vi "SQL查询.vi"(7 "condition":string, 8 "error in (no error)":errorcluster, 9 "columns":string[](array[string]), 10 "table输入":string(combo), 11 "database":string(combo)) -> (0 "error out":errorcluster, 1 "拆分数据":bool, 2 "columns输出":string[](array[string]), 3 "data":string[][](table))   [LabVIEW 2016, in "数据传输系统.lvlib"]
uses:
  <vilib>/Utility/sysdir.llb/System Directory Type.ctl
  <vilib>/addons/database/Connection.llb/DB Tools Open Connec (String).vi
  <vilib>/addons/database/_DB Variant To Data/Database Variant To Data.xnode
  <vilib>/addons/database/NI_Database_API.lvlib
panel:
  out "元素":string
  out "子数组":string[](array[string])
  # "时间 > #2021/01/15 08:00:00#and 时间 < #2021/04/15 08:00:00# order by 时间 asc"
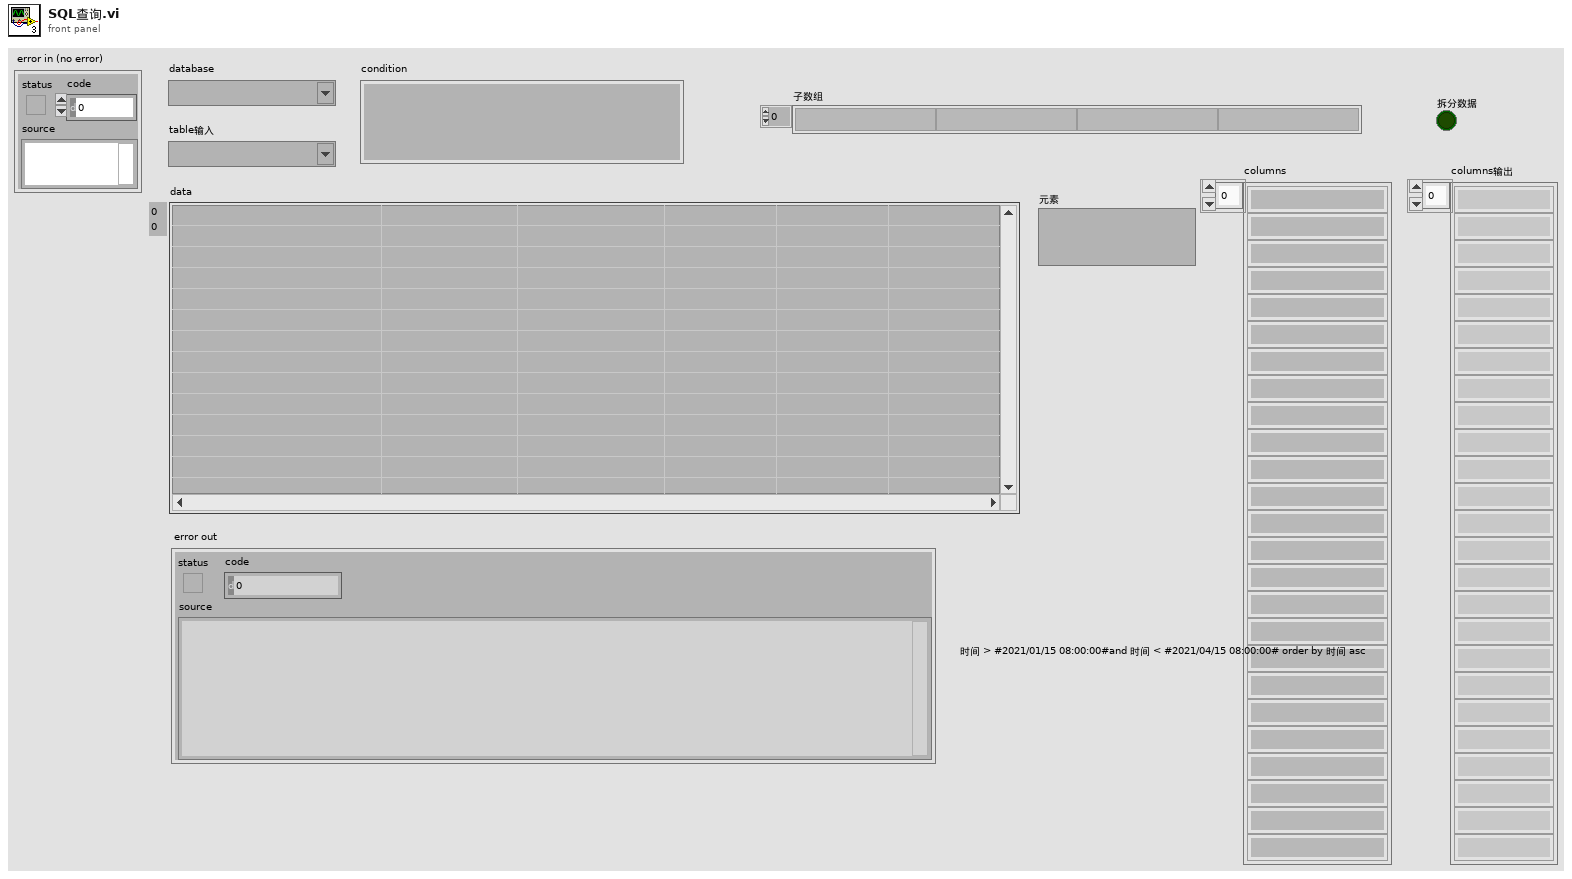
[diagram p1: front panel]
types:
  T1 = typedef "System Directory Type.ctl" = i32
  T2 = typedef "NI_Database_API.lvlib/Conn ObjectReference.ctl" = refnum<k1>
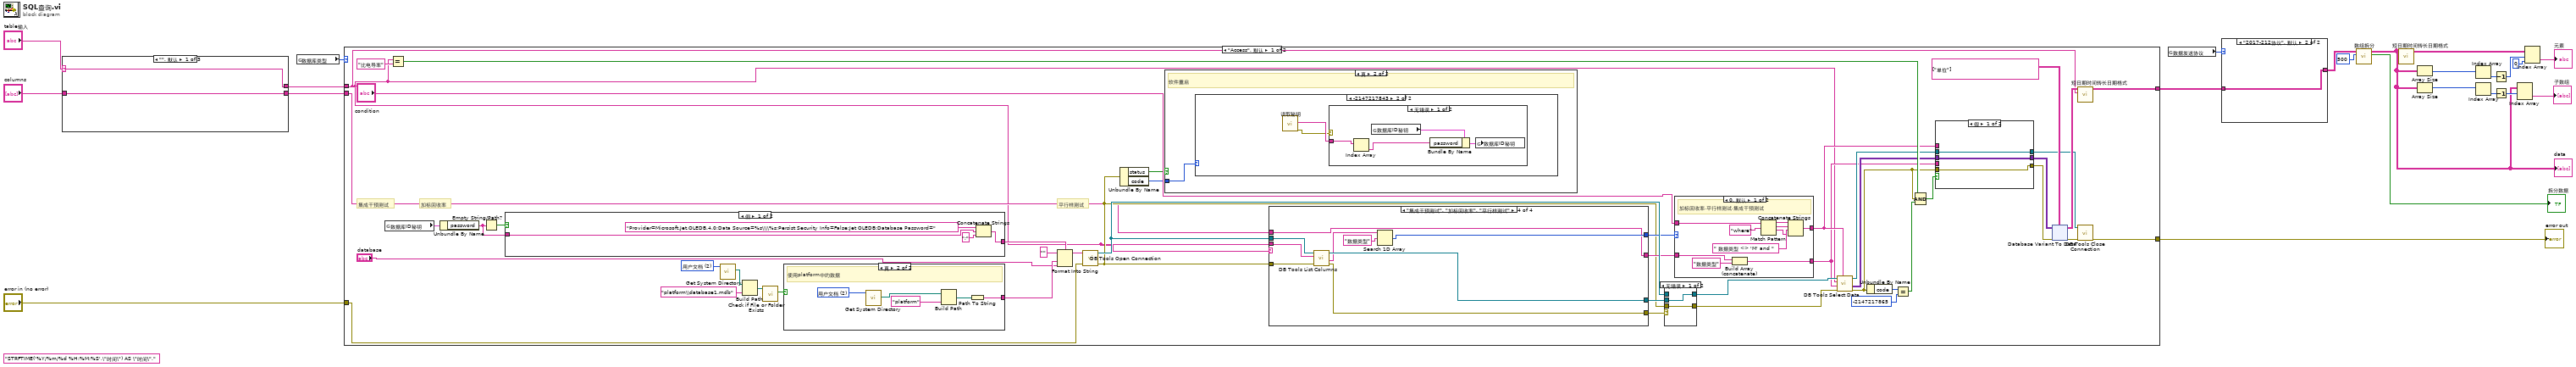
[diagram p0: block diagram]
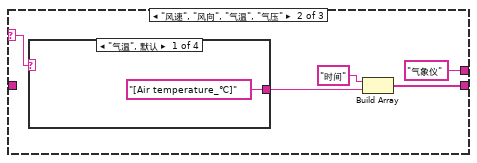
[diagram p2: hidden frame]
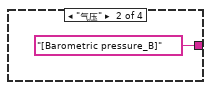
[diagram p3: hidden frame]
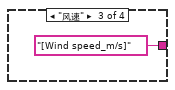
[diagram p4: hidden frame]
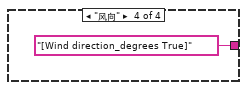
[diagram p5: hidden frame]
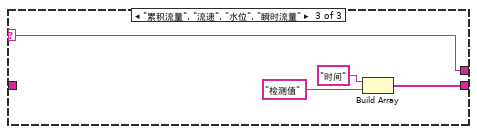
[diagram p6: hidden frame]
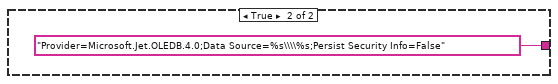
[diagram p7: hidden frame]
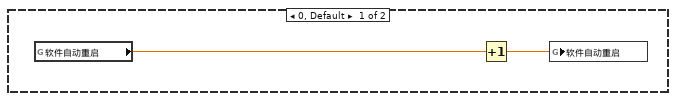
[diagram p9: hidden frame]
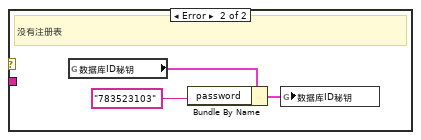
[diagram p10: hidden frame]
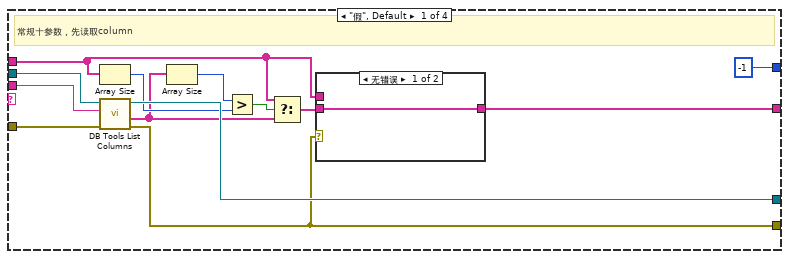
[diagram p13: hidden frame]
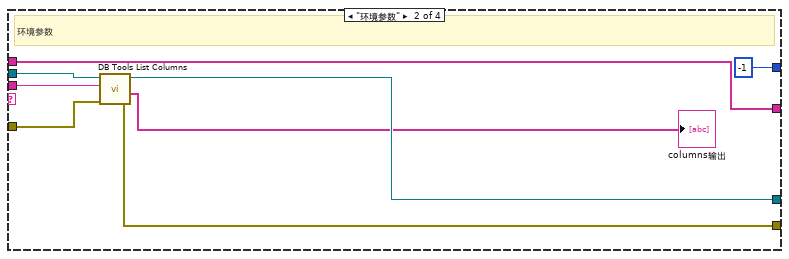
[diagram p15: hidden frame]
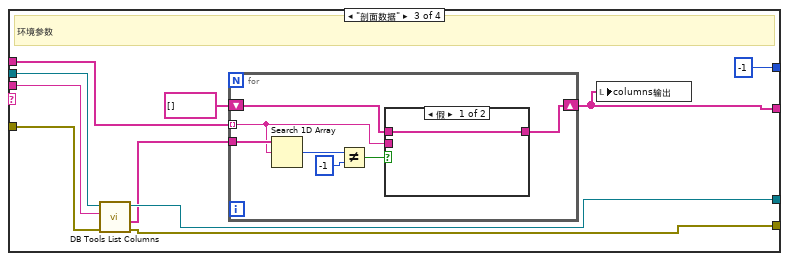
[diagram p16: hidden frame]
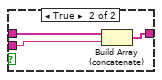
[diagram p17: hidden frame]
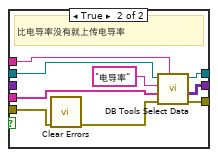
[diagram p18: hidden frame]
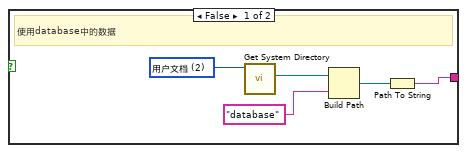
[diagram p19: hidden frame]
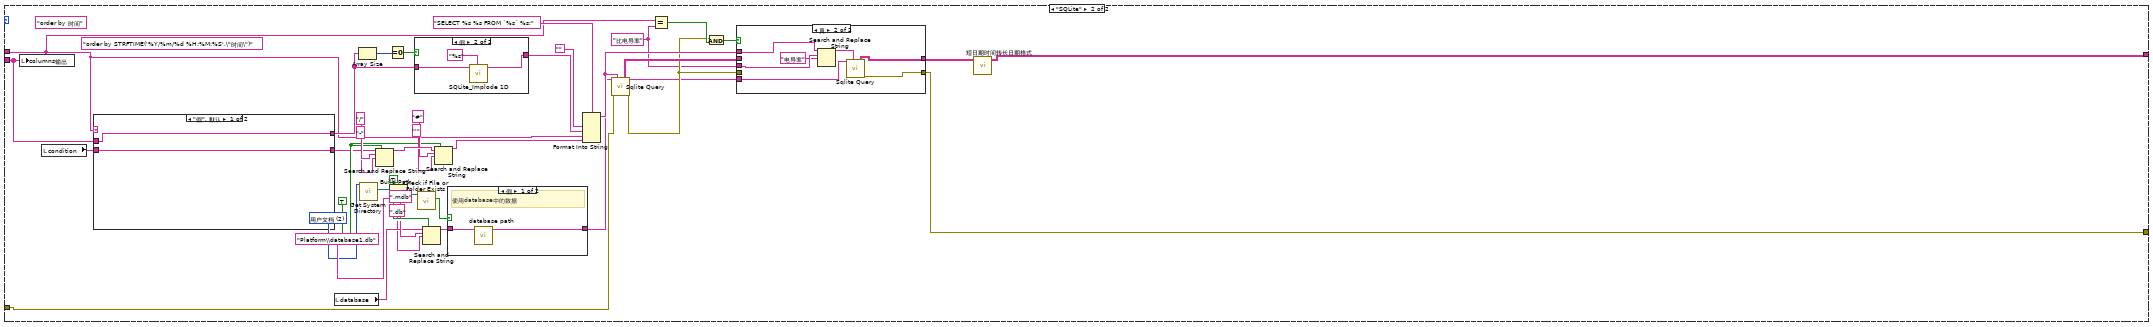
[diagram p20: hidden frame]
diagram:
  (unwired) "STRFTIME('%Y/%m/%d %H:%M:%S',\"时间\") AS \"时间\"," ("输入 1")
  n1 = case shown="\"\", 默认" "table输入" {
    selector: "table输入" -> [w25 w29 w35]
    tunnel: [w25 "气象仪" w35] -> w4
    tunnel: "columns" -> [w24 _ _]
    tunnel: [w24 w26 w37] -> w5
    frame "", Default {
    }
    frame "风速", "风向", "气温", "气压" {
      n2 = case shown="\"气温\", 默认" w29 {
        tunnel: ["[Air temperature_℃]" "[Barometric pressure_B]" "[Wind speed_m/s]" "[Wind direction_degrees True]"] -> w27
        frame "气温", Default {
        }
        frame "气压" {
        }
        frame "风速" {
        }
        frame "风向" {
        }
      }
      n3 = Build Array("时间", w27) -> (w26:string[])
    }
    frame "累积流量", "流速", "水位", "瞬时流量" {
      n4 = Build Array("时间", "检测值") -> (w37:string[])
    }
  }
  n5 = global read "断电保存全局.vi" "数据库类型"() -> (w8:enum16{"Access", "SQLite"})
  n6 = case shown="\"Access\", 默认" w8 {
    tunnel: [w79 w270] -> w23
    tunnel: [w51 w246] -> w11
    tunnel: "error in (no error)" -> [w43 w239]
    tunnel: w5 -> [w41 w242]
    tunnel: w4 -> [w40 w241]
    frame "Access", Default {
      w77 = T1 2 items=["用户目录"=0, "用户桌面"=1, "用户文档"=2, "用户应用程序数据"=3, "用户设置"=4, "用户临时目录"=5, "公共文档"=6, "公共应用程序数据"=7, "公共设置"=8, "公共缓存"=13, "系统核心库"=9, "系统安装库"=10, "应用程序文件"=11, "启动盘根目录"=12] ("system directory type")
      # "集成干预测试"
      # "平行样测试"
      # "加标回收率"
      n7 = global read "外部交互全局.vi" "数据库ID秘钥"() -> (w44:cluster{"userID":string, "password":string})
      n8 = Equal?(x=w40, y="比电导率") -> (x = y?=w71:bool)
      n9 = Unbundle By Name(w44) -> ("password"=w45:string)
      n10 = Empty String/Path?(string/path=w45) -> (empty?=w47:bool)
      n11 = case shown="假" w47 {
        tunnel: [w85 "Provider=Microsoft.Jet.OLEDB.4.0;Data Source=%s\\\\%s;Persist Security Info=False" ("格式字符串")] -> w46
        tunnel: w45 -> [w88 _]
        frame False {
          n12 = Concatenate Strings("Provider=Microsoft.Jet.OLEDB.4.0;Data Source=%s\\\\%s;Persist Security Info=False;Jet OLEDB:Database Password=" ("格式字符串"), w88, ";" ("字符串")) -> (w85:string)
        }
        frame True {
        }
      }
      n13 = call <vilib>:"Get System Directory.vi"("system directory type"=w77) -> ("system directory"=w78:path)  [unwired: 10 in]
      n14 = Build Path(base path=w78, name or relative path="platform\\database1.mdb" ("condition")) -> (appended path=w76:path)
      n15 = call <vilib>:"Check if File or Folder Exists.vi"("path"=w76) -> ("file or folder exists?"=w74:bool)  [unwired: 8 in, 2 out]
      n16 = case shown="真" w74 {
        tunnel: [w183 w188] -> w73
        frame False {
          w186 = T1 2 items=["用户目录"=0, "用户桌面"=1, "用户文档"=2, "用户应用程序数据"=3, "用户设置"=4, "用户临时目录"=5, "公共文档"=6, "公共应用程序数据"=7, "公共设置"=8, "公共缓存"=13, "系统核心库"=9, "系统安装库"=10, "应用程序文件"=11, "启动盘根目录"=12] ("system directory type")
          # "使用database中的数据"
          n17 = call <vilib>:"Get System Directory.vi"("system directory type"=w186) -> ("system directory"=w185:path)  [unwired: 10 in]
          n18 = Build Path(base path=w185, name or relative path="database" ("condition")) -> (appended path=w187:path)
          n19 = Path To String(path=w187) -> (string=w183:string)
        }
        frame True {
          w192 = T1 2 items=["用户目录"=0, "用户桌面"=1, "用户文档"=2, "用户应用程序数据"=3, "用户设置"=4, "用户临时目录"=5, "公共文档"=6, "公共应用程序数据"=7, "公共设置"=8, "公共缓存"=13, "系统核心库"=9, "系统安装库"=10, "应用程序文件"=11, "启动盘根目录"=12] ("system directory type")
          # "使用platform中的数据"
          n20 = call <vilib>:"Get System Directory.vi"("system directory type"=w192) -> ("system directory"=w191:path)  [unwired: 10 in]
          n21 = Build Path(base path=w191, name or relative path="platform" ("condition")) -> (appended path=w189:path)
          n22 = Path To String(path=w189) -> (string=w188:string)
        }
      }
      n23 = Format Into String(format string=w46, initial string="" ("初始字符串"), w73, "database") -> (resulting string=w81:string)  [unwired: 1 in, 1 out]
      n24 = call-poly <vilib>:"DB Tools Open Connection.vi"("error in (no error)"=w43, "connection information"=w81) -> ("error out"=w52:errorcluster, "connection reference"=w57:T2)  [unwired: 6 in]
      n25 = Unbundle By Name(w52) -> ("status"=w50:bool, "code"=w39:i32)
      n26 = case shown="真" w50 {
        tunnel: w39 -> [_ w90]
        frame False {
        }
        frame True {
          # "软件重启"
          n27 = case shown="-2147217843" w90 {
            frame 0, Default {
              n28 = global read "全局1.vi" "软件自动重启"() -> (w92:dbl)
              n29 = Increment(x=w92) -> (x+1=w91:dbl)
              n30 = global write "全局1.vi" "软件自动重启"(w91) -> ()
            }
            frame -2147217843 {
              n31 = call "读取秘钥.vi"() -> ("error out"=w93:errorcluster, "值"=w94:string[])  [unwired: 9 in, 1 out]
              n32 = case shown="无错误" w93 {
                tunnel: w94 -> [w98 _]
                frame No Error {
                  n33 = Index Array(array=w98) -> (element=w95:string)  [unwired: 1 in]
                  n34 = global read "外部交互全局.vi" "数据库ID秘钥"() -> (w96:cluster{"userID":string, "password":string})
                  n35 = Bundle By Name(cluster=w96, "password"=w95) -> (w97:cluster{"userID":string, "password":string})
                  n36 = global write "外部交互全局.vi" "数据库ID秘钥"(w97) -> ()
                }
                frame Error {
                  # "没有注册表"
                  n37 = global read "外部交互全局.vi" "数据库ID秘钥"() -> (w100:cluster{"userID":string, "password":string})
                  n38 = Bundle By Name(cluster=w100, "password"="783523103") -> (w101:cluster{"userID":string, "password":string})
                  n39 = global write "外部交互全局.vi" "数据库ID秘钥"(w101) -> ()
                }
              }
            }
          }
        }
      }
      n40 = case shown="\"集成干预测试\", \"加标回收率\", \"平行样测试\"" w40 {
        tunnel: w57 -> [w129 w140 w148 w170]
        tunnel: w52 -> [w126 w139 w147 w168]
        tunnel: [w127 w138 w145 w167] -> w59
        tunnel: [w121 w137 w146 w166] -> w60
        tunnel: w40 -> [w128 w136 w149 w169]
        tunnel: [-1 ("index of element") -1 ("index of element") -1 ("index of element") w163] -> w55
        tunnel: w41 -> [w118 w133 w144 w162]
        tunnel: [w119 w133 w141 w162] -> w53
        frame "假", Default {
          # "常规十参数，先读取column"
          n41 = Array Size(array=w118) -> (size(s)=w123:i32)
          n42 = call <vilib>:"DB Tools List Columns.vi"("error in (no error)"=w126, "table"=w128, "connection reference"=w129) -> ("error out"=w121:errorcluster, "columns"=w122:string[], "connection reference out"=w127:T2)  [unwired: 1 in, 1 out]
          n43 = Array Size(array=w122) -> (size(s)=w124:i32)
          n44 = Greater?(x=w124, y=w123) -> (0:w125:bool)
          n45 = Select(t=w118, s=w125, f=w122) -> (s? t:f=w120:string[])
          n46 = case shown="无错误" w121 {
            tunnel: w120 -> [w131 _]
            tunnel: [w131 w132] -> w119
            tunnel: w118 -> [_ w132]
            frame No Error {
            }
            frame Error {
            }
          }
        }
        frame "环境参数" {
          # "环境参数"
          n47 = call <vilib>:"DB Tools List Columns.vi"("error in (no error)"=w139, "table"=w136, "connection reference"=w140) -> ("error out"=w137:errorcluster, "columns"=→"columns输出":string[], "connection reference out"=w138:T2)  [unwired: 1 in, 1 out]
        }
        frame "剖面数据" {
          # "环境参数"
          n48 = call <vilib>:"DB Tools List Columns.vi"("error in (no error)"=w147, "table"=w149, "connection reference"=w148) -> ("error out"=w146:errorcluster, "columns"=w143:string[], "connection reference out"=w145:T2)  [unwired: 1 in, 1 out]
          n49 = for {
            tunnel: w144 -> [w153] mode=indexing
            tunnel: w143 -> [w157]
            shift-right: [w151] -> w141
            shift-left: string[] [] -> [w154]
            n50 = Search 1D Array(1D array=w157, element=w153) -> (index of element=w156:i32)  [unwired: 1 in]
            n51 = Not Equal?(x=w156, y=-1) -> (x != y?=w152:bool)
            n52 = case shown="假" w152 {
              tunnel: w154 -> [w158 w161]
              tunnel: w153 -> [_ w160]
              tunnel: [w158 w159] -> w151
              frame False {
              }
              frame True {
                n53 = Build Array (concatenate)(w161, w160) -> (w159:string[])
              }
            }
          }
          n54 = local write "columns输出"(w141) -> ()
        }
        frame "集成干预测试", "加标回收率", "平行样测试" {
          n55 = call <vilib>:"DB Tools List Columns.vi"("error in (no error)"=w168, "table"=w169, "connection reference"=w170) -> ("error out"=w166:errorcluster, "columns"=w165:string[], "connection reference out"=w167:T2)  [unwired: 1 in, 1 out]
          n56 = Search 1D Array(1D array=w165, element="数据类型" ("元素")) -> (index of element=w163:i32)  [unwired: 1 in]
        }
      }
      n57 = case shown="无错误" w60 {
        selector: w60 -> [_ w117]
        tunnel: w59 -> [w115 _]
        tunnel: [w115 w116] -> w58
        tunnel: w57 -> [_ w116]
        tunnel: [w114 w117] -> w56
        tunnel: w52 -> [w114 _]
        frame No Error {
        }
        frame Error {
        }
      }
      n58 = case "条件结构" shown="0, 默认" w55 {
        tunnel: "condition" -> [w109 w112]
        tunnel: w53 -> [w111 w113]
        tunnel: [w103 w113] -> w48
        tunnel: [w102 w112] -> w49
        frame 0, Default {
          # "加标回收率,平行样测试,集成干预测试"
          n59 = Build Array (concatenate)(w111, "数据类型" ("元素")) -> (w103:string[])
          n60 = Match Pattern(string=w109, regular expression="where" ("正则表达式")) -> (before substring=w107:string, match substring=w106:string, after substring=w104:string)  [unwired: 1 in, 1 out]
          n61 = Concatenate Strings(w107, w106, " 数据类型 <> 'M' and " ("字符串"), w104) -> (w102:string)
        }
        frame -1 {
        }
      }
      n62 = call <vilib>:"DB Tools Select Data.vi"("condition"=w49, "error in (no error)"=w56, "columns"=w48, "table"=w40, "connection reference"=w58) -> ("error out"=w64:errorcluster, "data"=w66:variant[][], "connection reference out"=w69:T2)  [unwired: 1 in]
      n63 = Unbundle By Name(w64) -> ("code"=w63:i32)
      n64 = Equal?(x=w63, y=-2147217865 ("code")) -> (x = y?=w61:bool)
      n65 = Compound Arithmetic op=AND ("复合运算")(w71, w64, w61) -> (w70:bool)
      n66 = case shown="假" w70 {
        tunnel: w49 -> [_ w182]
        tunnel: w69 -> [w173 w181]
        tunnel: [w173 w176] -> w68
        tunnel: [w172 w177] -> w67
        tunnel: w66 -> [w172 _]
        tunnel: w64 -> [w171 w179]
        tunnel: [w171 w175] -> w65
        tunnel: w48 -> [_ w174]
        frame False {
        }
        frame True {
          # "比电导率没有就上传电导率"
          n67 = call <vilib>:"Clear Errors.vi"("error in (no error)"=w179) -> ("error out"=w178:errorcluster)  [unwired: 5 in, 1 out]
          n68 = call <vilib>:"DB Tools Select Data.vi"("condition"=w182, "error in (no error)"=w178, "columns"=w174, "table"="电导率", "connection reference"=w181) -> ("error out"=w175:errorcluster, "data"=w177:variant[][], "connection reference out"=w176:T2)  [unwired: 1 in]
        }
      }
      n69 = xnode "Database Variant To Data"("database variant"=w67, "error in (no error)"=w65, "type"=string[][] [["单位"]]) -> ("data"=w80:string[][], "error out"=w82:errorcluster)
      n70 = call "短日期时间转长日期格式.vi"("table输入"=w40, "data"=w80) -> ("输出数组"=w79:string[][])  [unwired: 9 in]
      n71 = call <vilib>:"DB Tools Close Connection.vi"("error in (no error)"=w82, "connection reference"=w68) -> ("error out"=w51:errorcluster)  [unwired: 5 in]
    }
    frame "SQLite" {
      w244 = "比电导率" ("y")
      (unwired) "order by STRFTIME('%Y/%m/%d %H:%M:%S',\"时间\")" ("替换字符串(\"\")")
      (unwired) "order by 时间" ("搜索字符串")
      w255 = TRUE ("替换全部？(F)")
      w272 = T1 2 items=["用户目录"=0, "用户桌面"=1, "用户文档"=2, "用户应用程序数据"=3, "用户设置"=4, "用户临时目录"=5, "公共文档"=6, "公共应用程序数据"=7, "公共设置"=8, "公共缓存"=13, "系统核心库"=9, "系统安装库"=10, "应用程序文件"=11, "启动盘根目录"=12] ("system directory type")
      n72 = local write "columns输出"(w242) -> ()
      n73 = local read "condition"() -> (w254:string)
      n74 = case shown="\"假\", 默认" w241 {
        tunnel: w254 -> [w286 w292]
        tunnel: w242 -> [w285 w294]
        tunnel: [w285 w293] -> w265
        tunnel: [w286 w291] -> w253
        frame "假", Default {
        }
        frame "集成干预测试", "加标回收率", "平行样测试" {
          n75 = Build Array (concatenate)(w294, "数据类型" ("元素")) -> (w293:string[])
          n76 = call "数据库加密匹配 (子VI).vi"("输入参数"="N") -> ("Encoded String"=w289:string)  [unwired: 10 in]
          n77 = Match Pattern(string=w292, regular expression="where" ("正则表达式")) -> (before substring=w297:string, match substring=w296:string, after substring=w295:string)  [unwired: 1 in, 1 out]
          n78 = Format Into String(format string=" 数据类型 = '%s' and " ("字符串"), w289) -> (resulting string=w287:string)  [unwired: 2 in, 1 out]
          n79 = Concatenate Strings(w297, w296, w287, w295) -> (w291:string)
        }
      }
      n80 = local read "database"() -> (w257:string)
      n81 = Array Size(array=w265) -> (size(s)=w269:i32)
      n82 = call <vilib>:"Get System Directory.vi"("system directory type"=w272) -> ("system directory"=w271:path)  [unwired: 10 in]
      n83 = Search and Replace String(replace all?=w255, input string=w253, search string="/" ("搜索字符串"), replace string="-" ("替换字符串(\"\")")) -> (result string=w262:string)  [unwired: 4 in, 3 out]
      n84 = Equal To 0?(x=w269) -> (x = 0?=w268:bool)
      n85 = Build Path(base path=w271, name or relative path="Platform\\database1.db" ("condition")) -> (appended path=w273:path)
      n86 = case shown="假" w268 {
        tunnel: w265 -> [_ w302]
        tunnel: ["*" ("t") w301] -> w266
        frame True {
        }
        frame False {
          n87 = call <userlib>:"SQLite_Implode 1D.vi"("Values"=w302, "format string"="%s") -> ("imploded string"=w301:string)  [unwired: 7 in, 1 out]
        }
      }
      n88 = call <vilib>:"Check if File or Folder Exists.vi"("path"=w273) -> ("file or folder exists?"=w275:bool)  [unwired: 8 in, 2 out]
      n89 = Search and Replace String(replace all?=TRUE ("替换全部？(F)"), input string=w257, search string=".mdb" ("搜索字符串"), replace string=".db" ("替换字符串(\"\")")) -> (result string=w252:string)  [unwired: 4 in, 3 out]
      n90 = Search and Replace String(replace all?=w255, input string=w262, search string="#" ("搜索字符串"), replace string="'" ("替换字符串(\"\")")) -> (result string=w237:string)  [unwired: 4 in, 3 out]
      n91 = case shown="假" w275 {
        tunnel: [w305 w306] -> w240
        tunnel: w252 -> [w304 w307]
        frame False {
          # "使用database中的数据"
          n92 = call "database path.vi"("database"=w304) -> ("Path out"=w305:string)  [unwired: 9 in, 1 out]
        }
        frame True {
          # "使用platform中的数据"
          n93 = call "database platform path.vi"("database"=w307) -> ("Path out"=w306:string)  [unwired: 10 in]
        }
      }
      n94 = Format Into String(format string="SELECT %s %s FROM `%s` %s;" ("SQL Query"), "", w266, w241, w237) -> (resulting string=w247:string)  [unwired: 2 in, 1 out]
      n95 = call "Sqlite Query.vi"("DB Path"=w240, "SQL Query"=w247, "error in (no error)"=w239) -> ("Results"=w249:string[][], "DB Path Out"=w243:string, "error out"=w245:errorcluster)  [unwired: 10 in]
      n96 = Equal?(x=w241, y=w244) -> (x = y?=w251:bool)
      n97 = And(x=w245, y=w251) -> (x .and. y?=w250:bool)
      n98 = case shown="真" w250 {
        tunnel: w249 -> [w277 _]
        tunnel: [w277 w284] -> w248
        tunnel: w247 -> [_ w281]
        tunnel: w243 -> [_ w283]
        tunnel: [w276 w282] -> w246
        tunnel: w245 -> [w276 _]
        tunnel: w244 -> [_ w280]
        frame False {
        }
        frame True {
          n99 = Search and Replace String(input string=w281, search string=w280, replace string="电导率" ("Tables Name")) -> (result string=w278:string)  [unwired: 5 in, 3 out]
          n100 = call "Sqlite Query.vi"("DB Path"=w283, "SQL Query"=w278) -> ("Results"=w284:string[][], "error out"=w282:errorcluster)  [unwired: 11 in, 1 out]
        }
      }
      n101 = call "短日期时间转长日期格式.vi"("data"=w248) -> ("输出数组"=w270:string[][])  [unwired: 10 in]
    }
  }
  "error out" <- w11
  n102 = global read "断电保存全局.vi" "数据发送协议"() -> (w22:enum16{"2005-212协议", "2017-212协议"})
  n103 = case shown="\"2017-212协议\", 默认" w22 {
    tunnel: w23 -> [w309 w316]
    tunnel: [w308 w316] -> w9
    frame "2005-212协议" {
      n104 = for {
        N: 1 -> [_]
        tunnel: string[][] [] ("data") -> [w315]
        tunnel: w309 -> [w314] mode=indexing
        tunnel: [w312] -> w308
        n105 = Insert Into Array(array=w315, index (row)=0 ("索引 (行)"), new element=w314) -> (w312:string[][])  [unwired: 1 in]
      }
    }
    frame "2017-212协议", Default {
    }
  }
  n106 = call "数组拆分.vi"("拆分大小"=500, "输入数据"=w9) -> ("拆分数据"=→"拆分数据":bool, "输出数组"=w1:string[][])  [unwired: 8 in]
  "data" <- w1
  n107 = call "短日期时间转长日期格式.vi"("data"=w1) -> ("输出数组"=w17:string[][])  [unwired: 10 in]
  n108 = Array Size(array=w1) -> (size(s)=w16:i32[])
  n109 = Array Size(array=w1) -> (size(s)=w21:i32[])
  n110 = Index Array(array=w16) -> (element=w15:i32)  [unwired: 1 in]
  n111 = Index Array(array=w21) -> (element=w19:i32)  [unwired: 1 in]
  n112 = Decrement(x=w15) -> (x-1=w14:i32)
  n113 = Decrement(x=w19) -> (x-1=w18:i32)
  n114 = Index Array(array=w1, index (row)=w18) -> (element=→"子数组":string[])  [unwired: 1 in]
  n115 = Index Array(array=w17, index (row)=w14, index (col)=0 ("禁用的索引 (列)")) -> (element=→"元素":string)
